vi "tm_startrecorder.vi"(8 "error in (no error)":errorcluster, 9 "frames":i32, 10 "File":path, 11 "Handle in":u32) -> (0 "error out":errorcluster, 3 "Handle out":u32)   [LabVIEW 2015]
uses:
  tmcamcon.dll
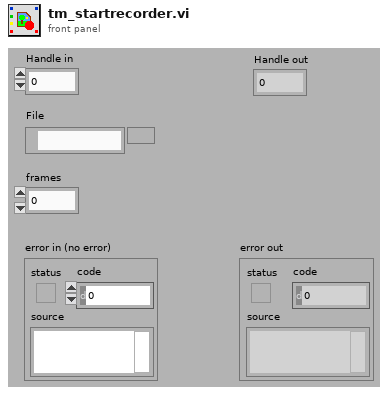
[diagram p1: front panel]
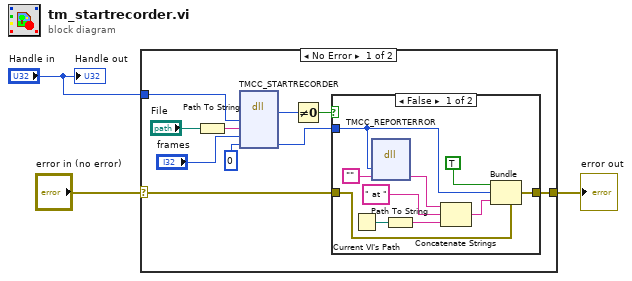
[diagram p0: block diagram]
diagram:
  n1 = case shown="No Error" "error in (no error)" {
    selector: "error in (no error)" -> [w11 w25]
    tunnel: [w8 w25] -> w2
    tunnel: "Handle in" -> [w7 _]
    frame No Error {
      n2 = Path To String(path="File") -> (string=w5:string)
      n3 = dll-call lib="tmcamcon.dll" fn="TMCC_STARTRECORDER"("handle"=w7, "path"=w5, "frames"="frames", "Erval"=0) -> ("return type"=w13:u32, "Erval"=w10:i32)  [unwired: 6 in, 2 out]
      n4 = Not Equal To 0?(x=w13) -> (x != 0?=w9:bool)
      n5 = case shown="False" w9 {
        tunnel: w11 -> [w23 w24]
        tunnel: [w22 w24] -> w8
        tunnel: w10 -> [w16 _]
        frame False {
          n6 = Current VI's Path() -> (path=w21:path)
          n7 = dll-call lib="tmcamcon.dll" fn="TMCC_REPORTERROR"("error"=w16, "buf"="") -> ("buf"=w15:string)  [unwired: 5 in, 2 out]
          n8 = Path To String(path=w21) -> (string=w17:string)
          n9 = Concatenate Strings(w15, " at ", w17) -> (w20:string)
          n10 = Bundle(cluster=w23, "status"=TRUE, "code"=w16, "source"=w20) -> (w22:errorcluster)
        }
        frame True {
        }
      }
    }
    frame Error {
    }
  }
  "error out" <- w2
  "Handle out" <- "Handle in"
